vi "startTest.vi"(8 "error in (no error)":errorcluster, 10 "model":refnum<class "Model.lvclass">, 11 "StoppedState in":refnum<class "StoppedState.lvclass">) -> (0 "error out":errorcluster, 2 "model 2":refnum<class "Model.lvclass">, 3 "StoppedState out":refnum<class "StoppedState.lvclass">)   [LabVIEW 2015, in "StoppedState.lvclass"]
uses:
  StoppedState.lvclass
  Model/Model/Model.lvclass
  Typedefs/StateSelector.ctl
  Typedefs/M1M3SSSTypedefs.lvlib
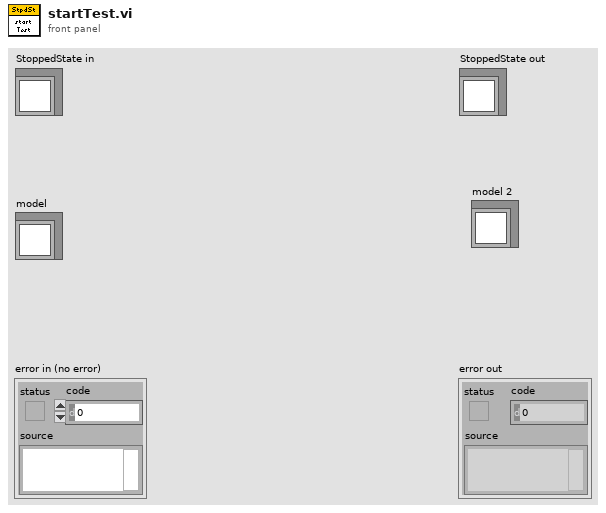
[diagram p1: front panel]
types:
  T1 = typedef "M1M3SSSTypedefs.lvlib/StateSelector.ctl" = enum16{"FaultState", "OffState", "RampingUpPressurePState", "RampingUpPressureSTState", "StandbyState", "StoppedState", "WaitingForSettledPState", "WaitingForSettledSTState"}
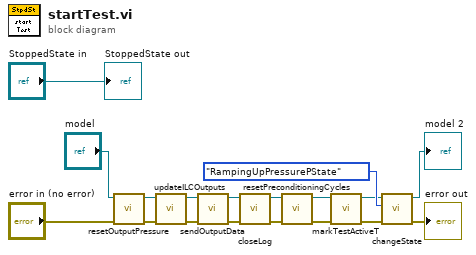
[diagram p0: block diagram]
diagram:
  n1 = call "resetOutputPressure.vi"("error in (no error)"="error in (no error)", "Model in"="model") -> ("error out"=w16:errorcluster, "Model out"=w18:refnum<class "Model.lvclass">)  [unwired: 8 in]
  n2 = call "updateILCOutputs.vi"("error in (no error)"=w16, "Model in"=w18) -> ("error out"=w15:errorcluster, "Model out"=w17:refnum<class "Model.lvclass">)  [unwired: 8 in]
  n3 = call "sendOutputData.vi"("error in (no error)"=w15, "Model in"=w17) -> ("error out"=w13:errorcluster, "Model out"=w14:refnum<class "Model.lvclass">)  [unwired: 8 in]
  n4 = call "closeLog.vi"("error in (no error)"=w13, "Model in"=w14) -> ("error out"=w5:errorcluster, "Model out"=w6:refnum<class "Model.lvclass">)  [unwired: 8 in]
  n5 = call "resetPreconditioningCycles.vi"("error in (no error)"=w5, "Model in"=w6) -> ("error out"=w2:errorcluster, "Model out"=w4:refnum<class "Model.lvclass">)  [unwired: 8 in]
  n6 = call "markTestActiveT.vi"("error in (no error)"=w2, "Model in"=w4) -> ("error out"=w1:errorcluster, "Model out"=w3:refnum<class "Model.lvclass">)  [unwired: 8 in]
  n7 = call "changeState.vi"("error in (no error)"=w1, "State:"=StateSelector."RampingUpPressurePState", "Model in"=w3) -> ("error out"=→"error out":errorcluster, "Model out"=→"model 2":refnum<class "Model.lvclass">)  [unwired: 7 in]
  "StoppedState out" <- "StoppedState in"
